vi "Set_Measurement_Conditions.vi"(0 "Traverse line":T6 {"Carrier_2 Q (l/min)" format="%#.2f"; "Row Duration (mins)" format="%#.1f"; "Row No" min=0; "Trace Gas Concentration (%)" min=0.0 format="%#_4f"; "Carrier_1 Q (l/min)" format="%#.4f"; "Start X" format="%#.2f"; "Start Y" format="%#.2f"; "Start Z" format="%#.2f"; "End X" format="%#.2f"; "End Y" format="%#.2f"; "End Z" format="%#.2f"; "Tunnel Speed" format="%#.2f"; "Averaging time (mins)" min=0.0 format="%#.2f"}, 1 "Gas Line Name":T1, 2 "Currently on Point":i32=11, 3 "Simulate/Run":T4, 4 "Source Establishment Time (s)":dbl=20.0) -> (7 "Status Cluster":T2)   [LabVIEW 2021]
uses:
  Traverse_cluster.ctl
  Spacing.ctl
  Controls/Multi_run_mode.ctl
  Execute_case.ctl
  Controls/User_Specific_mode.ctl
  Status_Cluster.ctl
  Multi_Run_Status.ctl
  Controls/GMU Gas Line Name.ctl
  ADAM Client/Sub VIs/ADAM Controls/Client_Source_Status.ctl
  Globals/Preference_global.vi
  Globals/Extra_Commands_Global.vi
panel:
  out "Heaters On?":bool
  out "Time Source Started":dbl
  out "Execute Case":T5=enum."Set All Conditions"
  # "X           Y          Z"
  # "Start"
  # "End"
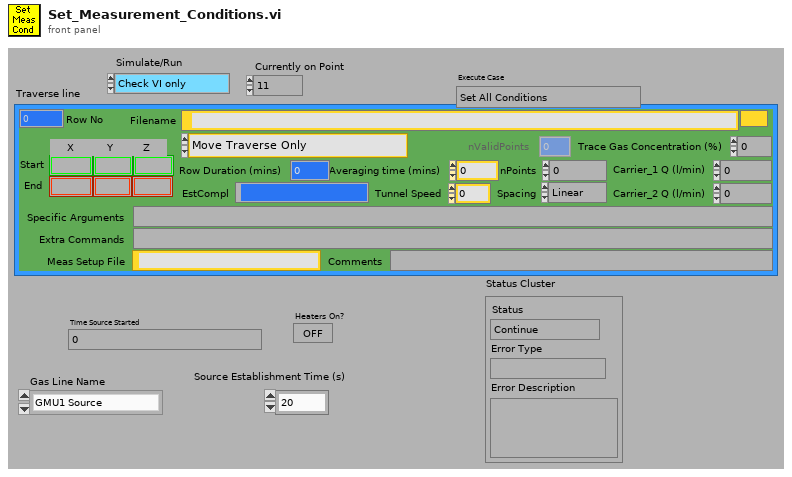
[diagram p1: front panel]
types:
  T1 = typedef "GMU Gas Line Name.ctl" = enum16{"GMU1 Source", "GMU2 Source", "GMU2 Calib", "CPP GRC-A", "CPP GRC-B"}
  T2 = typedef "Status_Cluster.ctl" = cluster{"Status":T3, "Error Type":string, "Error Description":string}
  T3 = typedef "Multi_Run_Status.ctl" = enum16{"Continue", "Continue with Error", "Jump to Next Point", "Jump to Next Row", "Jump To Fall Back", "Terminate Run"}
  T4 = typedef "User_Specific_mode.ctl" = enum16{"Check VI only", "Run VI"}
  T5 = typedef "Execute_case.ctl" = enum16{"Start", "EnFlo Tunnel Check", "Set All Conditions", "Establish Exp Conditions", "The End"}
  T6 = typedef "Traverse_cluster.ctl" = cluster{"Start X":sgl, "Start Y":sgl, "Start Z":sgl, "End X":sgl, "End Y":sgl, "End Z":sgl, "nPoints":i32, "Spacing":T7, "Filename":path, "Tunnel Speed":dbl, "Averaging time (mins)":dbl, "Extra Commands":string, "Carrier_1 Q (l/min)":dbl, "Carrier_2 Q (l/min)":dbl, "Trace Gas Concentration (%)":dbl, "Specific Arguments":string, "Comments":string, "Row No":i32, "Row Type Selector":T8, "EstCompl":string, "Row Duration (mins)":dbl, "nValidPoints":i32, "Meas Setup File":string}
  T7 = typedef "Spacing.ctl" = enum16{"Linear", "Log", "Gauss", "Specified", "N/A"}
  T8 = typedef "Multi_run_mode.ctl" = enum16{"Move Traverse Only", "Set Tunnel Speed Only", "Set Source Only", "Set Measurement Conditions", "Single Measurement", "Vertical Profile", "Lateral Profile", "Longitudinal Profile", "Multi-Axis Profile", "Explore Volume", "Auto Calibrate", "Meas Fast FID Bkgnd", "Check Beam Power", "Scanning Valve Measurement", "Run VI Named:", "Set ADAM Ch", "Wait (minutes)", "Send Message", "Synchronize With:", "Fall Back to this Row", "Turn Off Row Repeating", "Traverse 3D Volume", "Blank Row", "Jump to Fall Back Row"}
  T9 = typedef "Client_Source_Status.ctl" = enum16{"Not Using", "Using", "Must Have"}
  T10 = typedef "Server_Comms.ctl" = enum16{"Do Not Link To Server", "Server Link Healthy"}
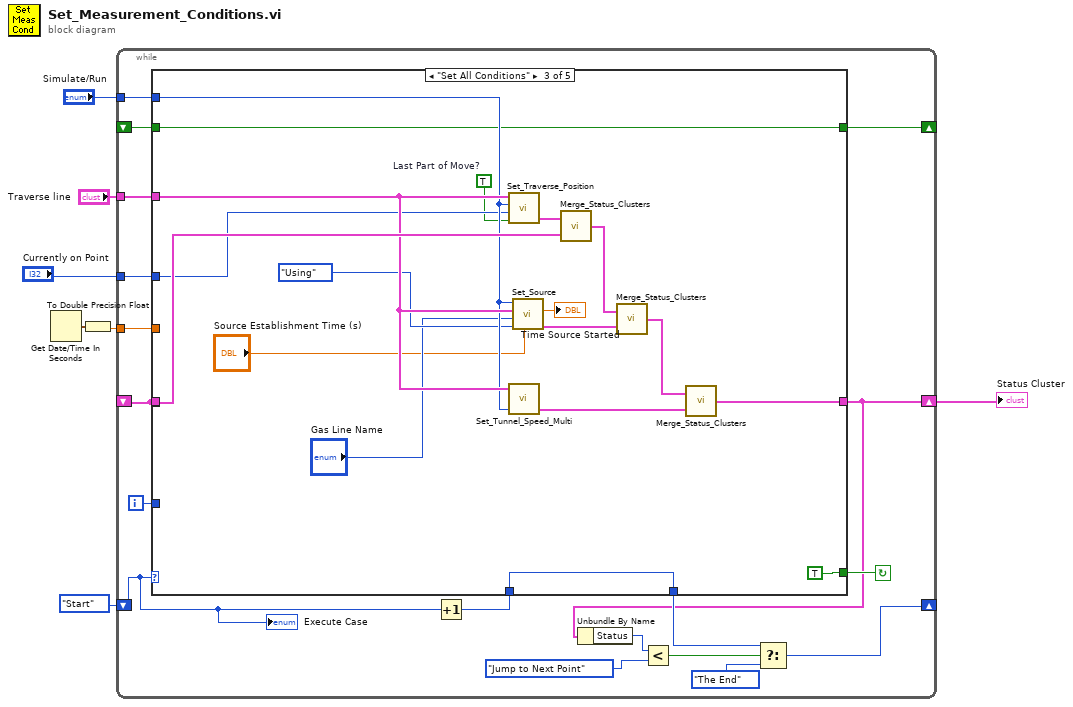
[diagram p0: block diagram]
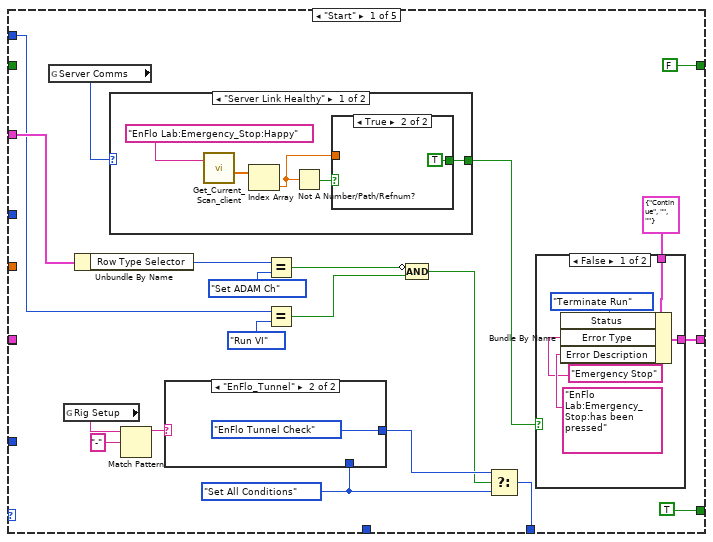
[diagram p2: hidden frame]
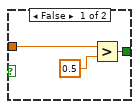
[diagram p4: hidden frame]
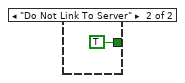
[diagram p5: hidden frame]
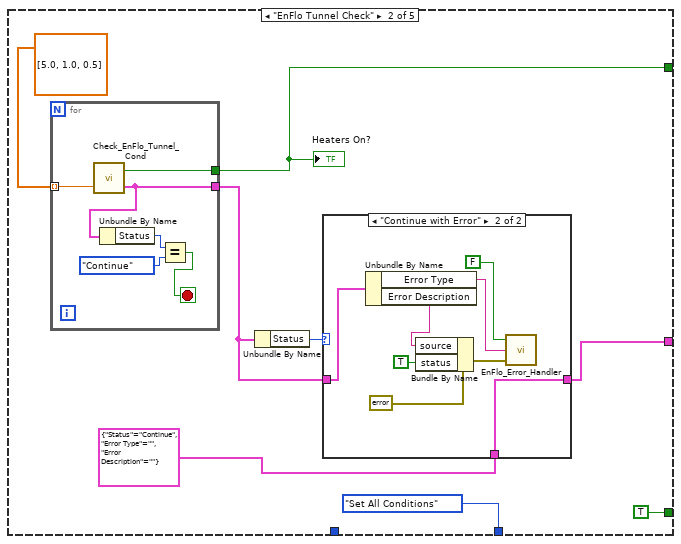
[diagram p7: hidden frame]
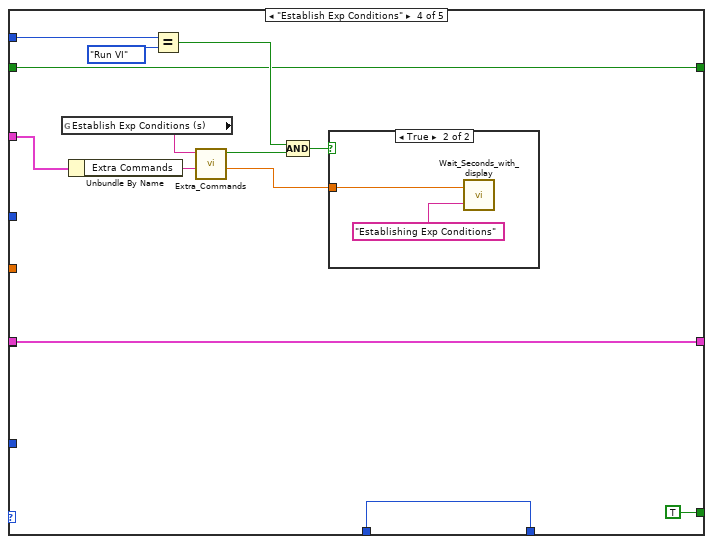
[diagram p9: hidden frame]
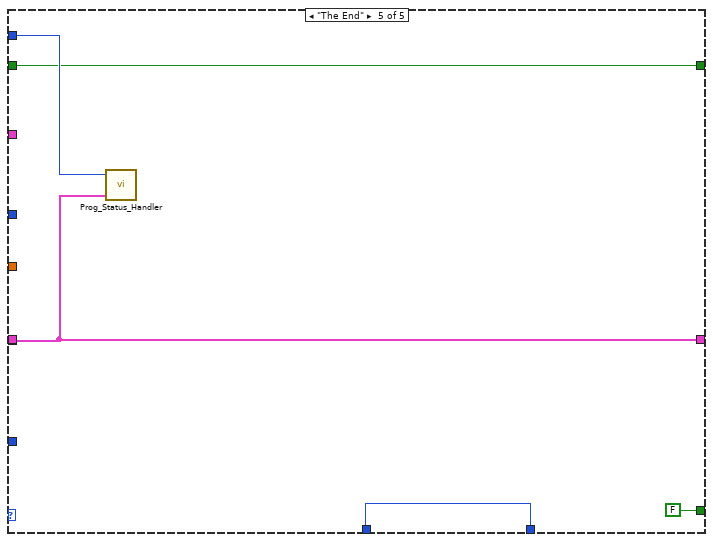
[diagram p11: hidden frame]
diagram:
  n1 = Get Date/Time In Seconds() -> (seconds since 1Jan1904=w1:timestamp)
  n2 = To Double Precision Float(number=w1) -> (double precision float=w2:dbl)
  n3 = while {
    tunnel: w2 -> [w15]
    tunnel: "Traverse line" -> [w16]
    tunnel: "Currently on Point" -> [w17]
    shift-left: _ -> [w18]
    shift-right: [w11] -> w4
    tunnel: "Simulate/Run" -> [w22]
    shift-left: Execute_case."Start" ("Execute Case") -> [w23]
    shift-right: [w20] -> _
    shift-right: [w13] -> _
    shift-left: _ -> [w12]
    i -> [w14]
    stop <- w25 continue-if-true
    n4 = Increment(x=w23) -> (x+1=w24:T5)
    n5 = case shown="\"Set All Conditions\"" w23 {
      tunnel: [TRUE TRUE TRUE TRUE FALSE] -> w25
      tunnel: w24 -> [_ _ w99 w108 w123]
      tunnel: w22 -> [w43 _ w97 w116 w122]
      tunnel: w18 -> [_ _ w103 w107 w120]
      tunnel: [w27 w67 w100 w107 w120] -> w11
      tunnel: [w40 Execute_case."Set All Conditions" ("Execute Case") w99 w108 w123] -> w19
      tunnel: w18 -> [_ _ _ _ _]
      tunnel: w17 -> [_ _ w96 _ _]
      tunnel: w16 -> [w45 _ w102 w115 _]
      tunnel: w15 -> [_ _ _ _ _]
      tunnel: w14 -> [_ _ _ _ _]
      tunnel: [FALSE w69 w93 w106 w121] -> w13
      tunnel: w12 -> [_ _ w93 w106 w121]
      frame "Start" {
        w41 = Execute_case."Set All Conditions" ("Execute Case")
        n6 = global read "Preference_global.vi" "Server Comms"() -> (w30:T10)
        n7 = global read "Preference_global.vi" "Rig Setup"() -> (w33:string)
        n8 = Unbundle By Name(w45) -> ("Row Type Selector"=w35:T8)
        n9 = case shown="\"Server Link Healthy\"" w30 {
          tunnel: [w53 TRUE] -> w29
          frame "Server Link Healthy" {
            n10 = call "Get_Current_Scan_client.vi"("singleChannel"="EnFlo Lab:Emergency_Stop:Happy") -> ("Numerical Values"=w56:dbl[])  [unwired: 1 in, 3 out]
            n11 = Index Array(array=w56) -> (element=w54:dbl)  [unwired: 1 in]
            n12 = Not A Number/Path/Refnum?(number/path/refnum=w54) -> (NaN/Path/Refnum?=w55:bool)
            n13 = case shown="True" w55 {
              tunnel: w54 -> [w59 _]
              tunnel: [w57 TRUE] -> w53
              frame False {
                n14 = Greater?(x=w59, y=0.5) -> (0:w57:bool)
              }
              frame True {
              }
            }
          }
          frame "Do Not Link To Server" {
          }
        }
        n15 = Match Pattern(string=w33, regular expression="-") -> (before substring=w32:string)  [unwired: 4 out]
        n16 = case shown="\"EnFlo_Tunnel\"" w32 {
          tunnel: [w62 Execute_case."EnFlo Tunnel Check" ("Execute Case")] -> w42
          tunnel: w41 -> [w62 _]
          frame "Other", Default {
          }
          frame "EnFlo_Tunnel" {
          }
        }
        n17 = Equal?(x=w35, y=Multi_run_mode."Set ADAM Ch" ("Mode")) -> (x = y?=w38:bool)
        n18 = Equal?(x=w43, y=User_Specific_mode."Run VI" ("Simulate/Run")) -> (x = y?=w37:bool)
        n19 = Compound Arithmetic op=AND(invert w38, w37) -> (w36:bool)
        n20 = Select(t=w42, s=w36, f=w41) -> (s? t:f=w40:T5)
        n21 = case shown="False" w29 {
          tunnel: T2 {"Status"=enum."Continue", "Error Type"="", "Error Description"=""} ("Status Cluster") -> [w50 w51]
          tunnel: [w49 w51] -> w27
          frame False {
            n22 = Bundle By Name(cluster=w50, "Status"=Multi_Run_Status."Terminate Run", "Error Type"="Emergency Stop", "Error Description"="EnFlo Lab:Emergency_Stop:has been pressed") -> (w49:T2)
          }
          frame True {
          }
        }
      }
      frame "EnFlo Tunnel Check" {
        n23 = for {
          tunnel: [w77] -> w69
          tunnel: [w76] -> w66
          tunnel: dbl[] [5.0, 1.0, 0.5] -> [w75] mode=indexing
          stop <- w72 stop-if-true
          n24 = call "Check_EnFlo_Tunnel_Cond.vi"("Averaging time (mins)"=w75) -> ("Status Cluster"=w76:T2, "Heaters On?"=w77:bool)  [unwired: 1 in]
          n25 = Unbundle By Name(w76) -> ("Status"=w73:T3)
          n26 = Equal?(x=w73, y=Multi_Run_Status."Continue" ("Status")) -> (x = y?=w72:bool)
        }
        "Heaters On?" <- w69
        n27 = Unbundle By Name(w66) -> ("Status"=w68:T3)
        n28 = case shown="\"Continue with Error\"" w68 {
          tunnel: [w78 w86] -> w67
          tunnel: w66 -> [w78 w85]
          tunnel: T2 {"Status"=enum."Continue", "Error Type"="", "Error Description"=""} ("Status Cluster In") -> [_ w86]
          frame Default {
          }
          frame "Continue with Error" {
            n29 = Unbundle By Name(w85) -> ("Error Type"=w80:string, "Error Description"=w81:string)
            n30 = Bundle By Name(cluster=errorcluster {"status"=FALSE, "code"=0, "source"=""} ("error in (no error)"), "source"=w81, "status"=TRUE) -> (w83:errorcluster)
            n31 = call "EnFlo_Error_Handler.vi"("error in (no error)"=w83, "Error Type"=w80, "Dialog Box (F)"=FALSE ("Dialog Box (T)")) -> ()  [unwired: 1 in, 2 out]
          }
        }
      }
      frame "Set All Conditions" {
        w89 = TRUE  # Last Part of Move?
        n32 = call "Set_Traverse_Position.vi"("Last Part of Move?"=w89, "Currently on Point"=w96, "Simulate/Run"=w97, "Traverse line"=w102) -> ("Status Cluster"=w90:T2)  [unwired: 2 in]
        n33 = call "Set_Tunnel_Speed_Multi.vi"("Simulate/Run"=w97, "Traverse line"=w102) -> ("Status Cluster"=w101:T2)  [unwired: 3 out]
        n34 = call "Set_Source.vi"("Source Establishment Time (s)"="Source Establishment Time (s)", "Source Status"=Client_Source_Status."Using", "Gas Line Name"="Gas Line Name", "Traverse line"=w102, "Simulate/Run"=w97) -> ("Status Cluster"=w91:T2, "Time Source Started"=→"Time Source Started":dbl)  [unwired: 4 out]
        n35 = call "Merge_Status_Clusters.vi"("Status Cluster 2"=w103, "Status Cluster 1"=w90) -> ("Status Cluster Out"=w95:T2)
        n36 = call "Merge_Status_Clusters.vi"("Status Cluster 2"=w91, "Status Cluster 1"=w95) -> ("Status Cluster Out"=w94:T2)
        n37 = call "Merge_Status_Clusters.vi"("Status Cluster 2"=w101, "Status Cluster 1"=w94) -> ("Status Cluster Out"=w100:T2)
      }
      frame "Establish Exp Conditions" {
        n38 = global read "Extra_Commands_Global.vi" "Establish Exp Conditions (s)"() -> (w114:string)
        n39 = Unbundle By Name(w115) -> ("Extra Commands"=w109:string)
        n40 = Equal?(x=w116, y=User_Specific_mode."Run VI" ("Simulate/Run")) -> (x = y?=w110:bool)
        n41 = call "Extra_Commands.vi"("String to Search"=w109, "Command"=w114) -> ("Numeric Value"=w105:dbl, "Command Found"=w111:bool)  [unwired: 1 in, 3 out]
        n42 = Compound Arithmetic op=AND(w110, w111) -> (w112:bool)
        n43 = case shown="True" w112 {
          tunnel: w105 -> [_ w118]
          frame False {
          }
          frame True {
            n44 = call "Wait_Seconds_with_display.vi"("Message"="Establishing Exp Conditions", "Seconds to wait"=w118) -> ()  [unwired: 2 out]
          }
        }
      }
      frame "The End" {
        n45 = call "Prog_Status_Handler.vi"("Status Cluster"=w120, "Simulate/Run"=w122) -> ()  [unwired: 2 out]
      }
    }
    n46 = Unbundle By Name(w11) -> ("Status"=w10:T3)
    n47 = Less?(x=w10, y=Multi_Run_Status."Jump to Next Point" ("Status")) -> (x < y?=w8:bool)
    n48 = Select(t=w19, s=w8, f=Execute_case."The End" ("Execute Case")) -> (s? t:f=w20:T5)
    "Execute Case" <- w23
  }
  "Status Cluster" <- w4
